vi "main.vi"() -> ()   [LabVIEW 2022 SP3]
uses:
  message.ctl
  states.ctl
  operationTypes.ctl
  consumer_data_structure.ctl
  <vilib>/picture/picture.llb/imagedata.ctl
  <vilib>/picture/picture.llb/Draw True-Color Pixmap.vi
panel:
  in  "Sharpen":bool
  in  "Filter":bool
  in  "Blur":bool
  out "Processed image":picture
  out "Input image":picture
  in  "stop":bool
  in  "Image path":path
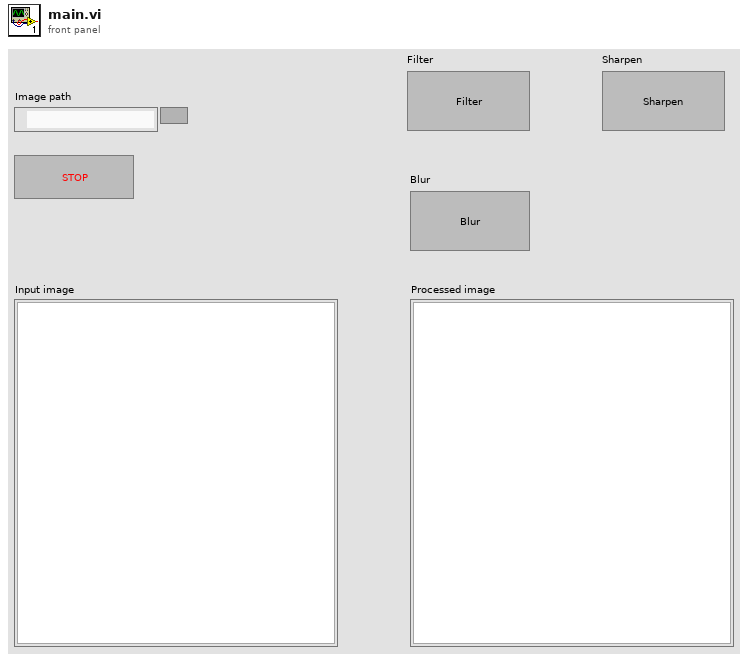
[diagram p1: front panel]
types:
  T1 = typedef "message.ctl" = cluster{"Command":T2, "data":variant}
  T2 = typedef "states.ctl" = enum16{"ErrorDefault", "Init", "ReadImage", "ProcessImage", "Stop"}
  T3 = typedef "operationTypes.ctl" = enum16{"Blur", "Sharpen", "Filter"}
  T4 = typedef "imagedata.ctl" = cluster{"image type":i32, "image depth":i32, "image":u8[], "mask":u8[], "colors":u32[], "Rectangle":cluster{"left":i16, "top":i16, "right":i16, "bottom":i16}}
  T5 = typedef "consumer_data_structure.ctl" = cluster{"Processed image":T4, "Input image":T4}
  T6 = typedef "LVBoundsTypeDef.ctl" = cluster{"Width":u32, "Height":u32}
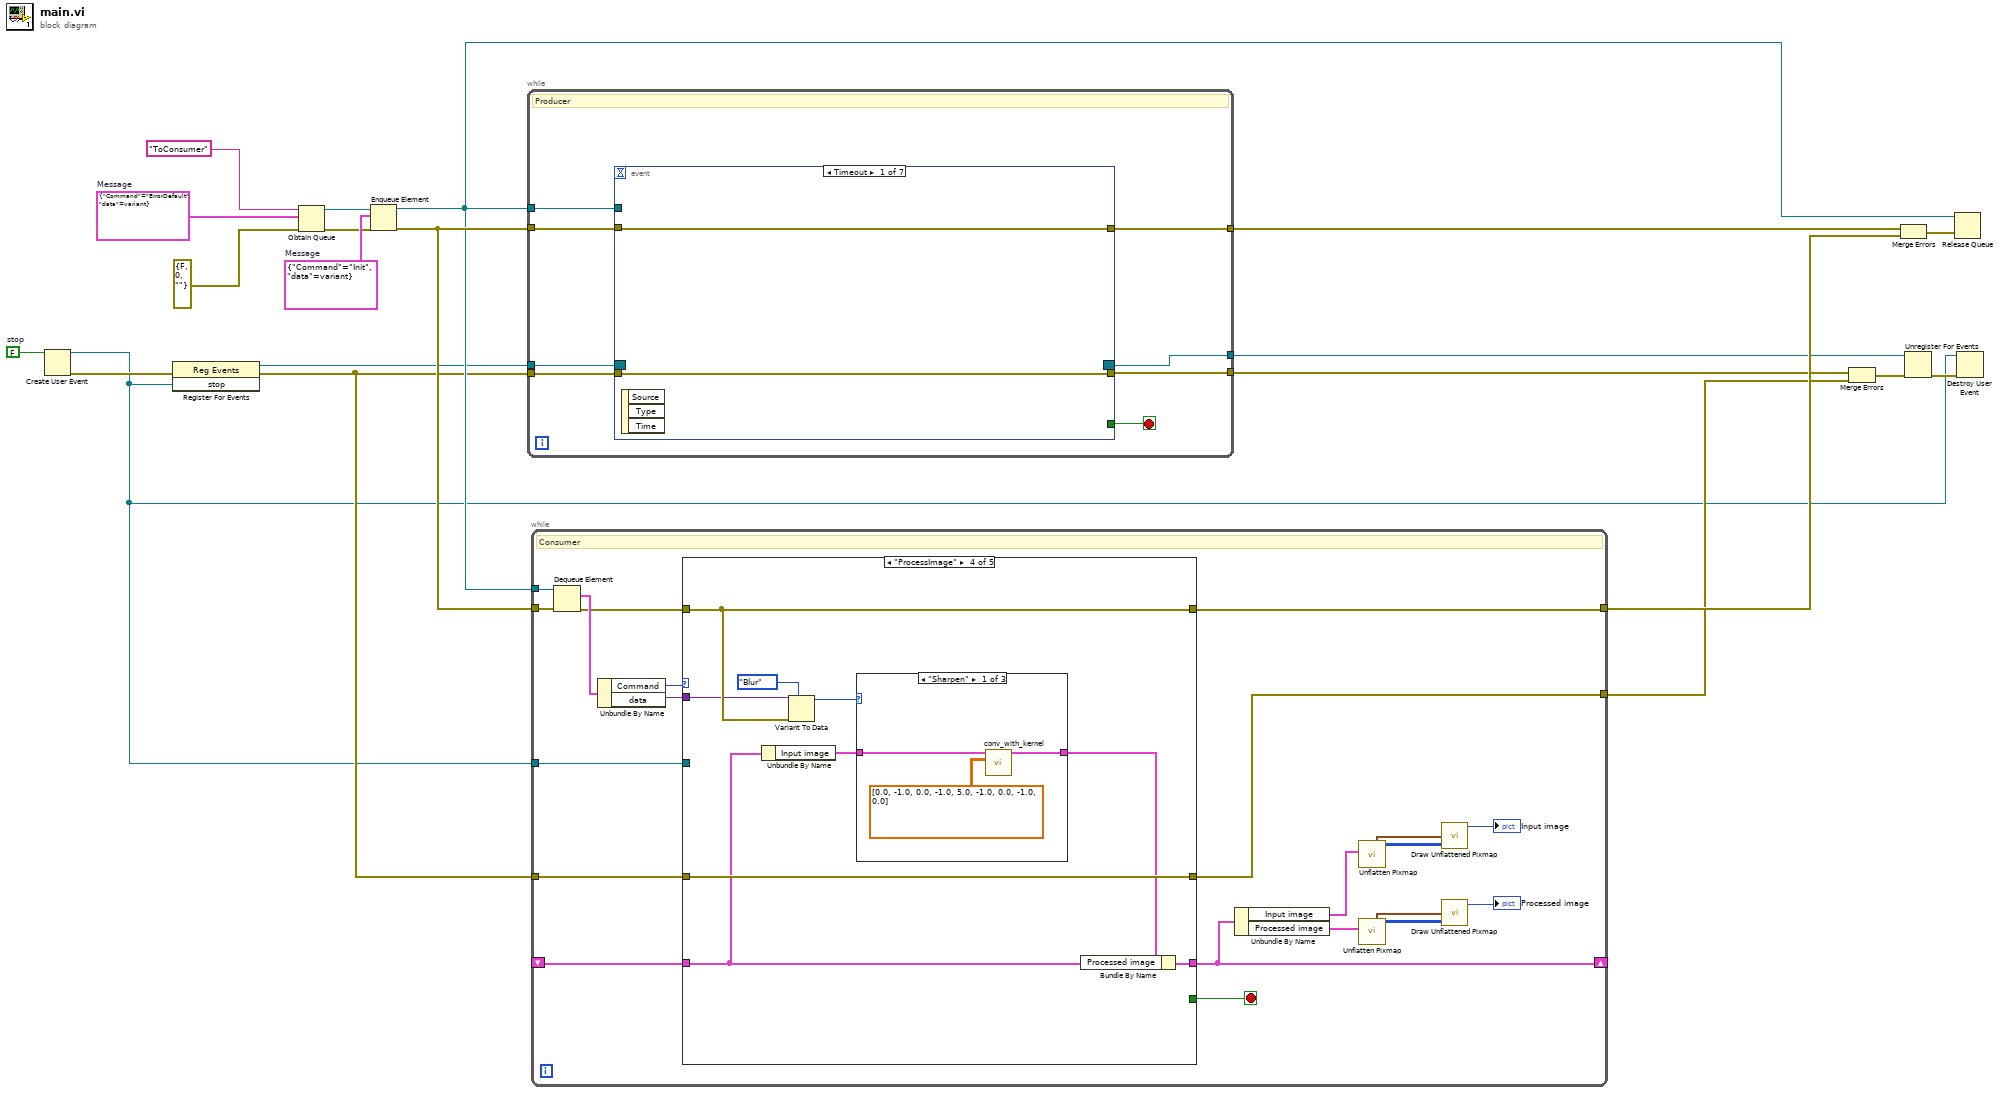
[diagram p0: block diagram]
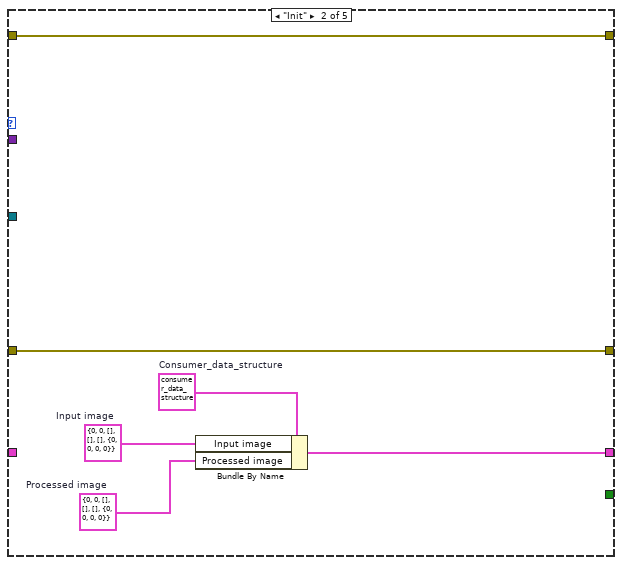
[diagram p3: hidden frame]
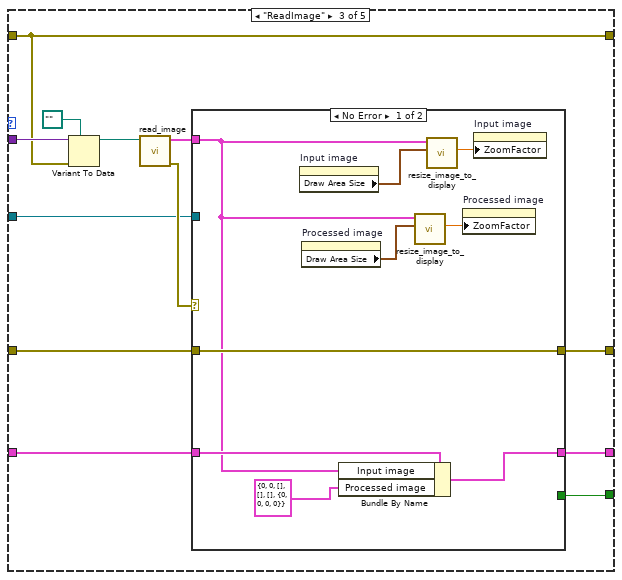
[diagram p4: hidden frame]
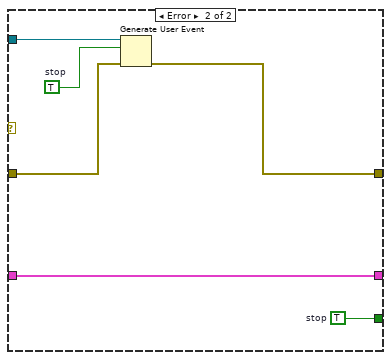
[diagram p5: hidden frame]
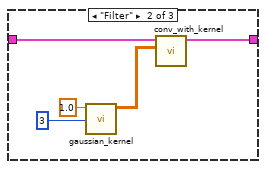
[diagram p6: hidden frame]
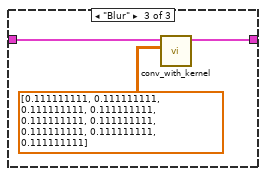
[diagram p7: hidden frame]
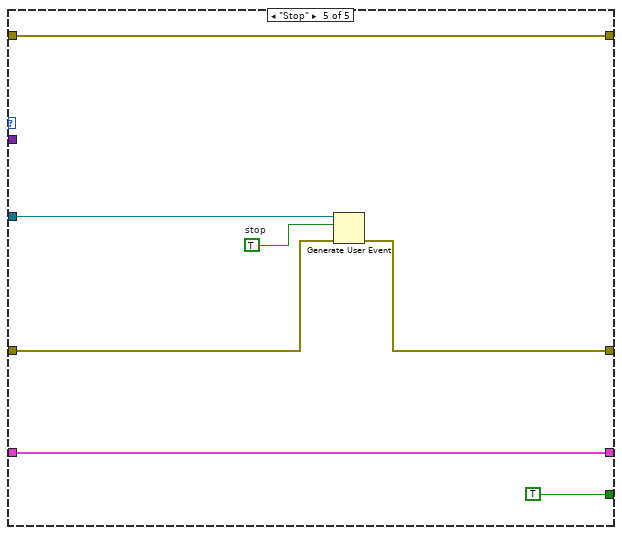
[diagram p8: hidden frame]
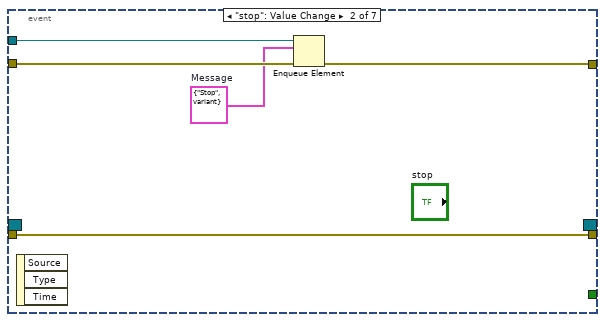
[diagram p9: hidden frame]
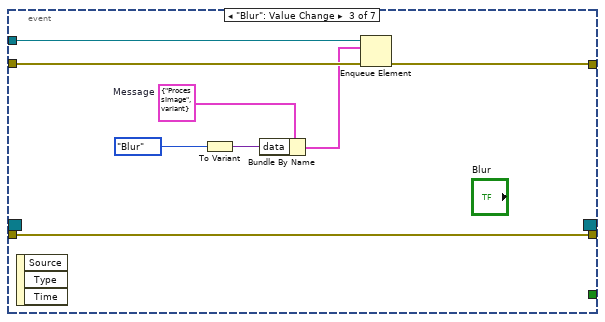
[diagram p10: hidden frame]
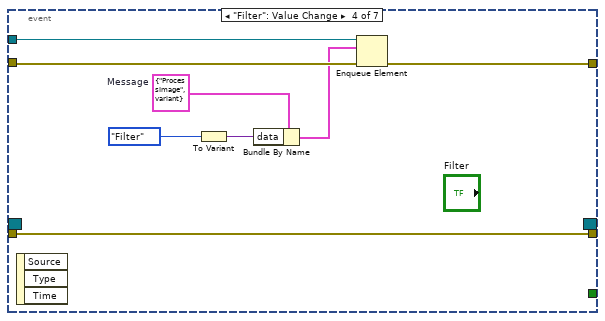
[diagram p11: hidden frame]
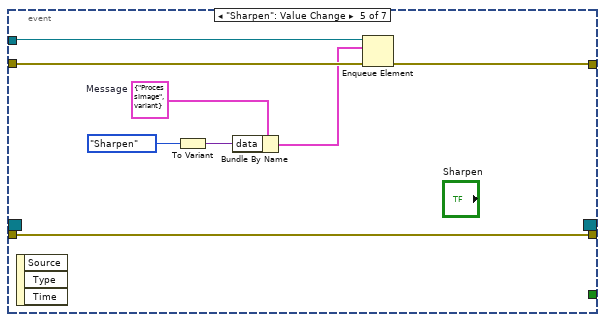
[diagram p12: hidden frame]
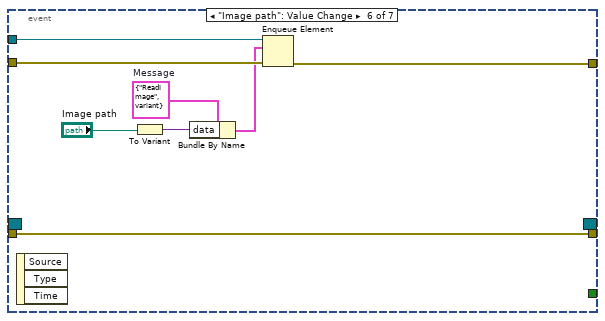
[diagram p13: hidden frame]
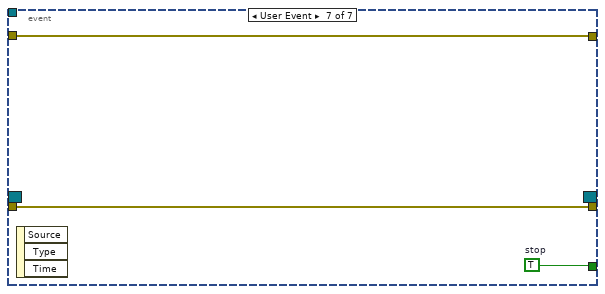
[diagram p14: hidden frame]
diagram:
  w10 = FALSE  # stop
  w18 = T1 {"Command"=enum."Init", "data"=variant(cluster{"Image path":path} {"Image path"=path ""})}  # Message
  w20 = T1 {"Command"=enum."ErrorDefault", "data"=variant(cluster{"Image path":path} {"Image path"=path ""})}  # Message
  n1 = Create User Event(user event datatype=w10) -> (user event=w1:refnum<user-event>, error out=w9:errorcluster)  [unwired: 1 in]
  n2 = register-events(error in=w9, w1) -> (reference out=w8:refnum<event-registration>, error out=w4:errorcluster)  [unwired: 1 in]
  n3 = Obtain Queue(name (unnamed)="ToConsumer", element data type=w20, error in (no error)=errorcluster {"status"=FALSE, "code"=0, "source"=""}) -> (queue out=w19:refnum<queue>, error out=w16:errorcluster)  [unwired: 2 in, 1 out]
  n4 = Enqueue Element(queue=w19, element=w18, error in (no error)=w16) -> (queue out=w11:refnum<queue>, error out=w15:errorcluster)  [unwired: 1 in, 1 out]
  n5 = while "Producer" {
    tunnel: w11 -> [w29]
    tunnel: w15 -> [w28]
    tunnel: [w27] -> w13
    tunnel: w8 -> [w25]
    tunnel: [w24] -> w6
    tunnel: w4 -> [w23]
    tunnel: [w22] -> w2
    stop <- w26 stop-if-true
    # "Producer"
    n6 = event shown="[0] Timeout" {
      selector: w25 -> [_ _ _ _ _ _ _]
      dyn-events: [_ _ _ _ _ _ _] -> w24
      timeout: _ -> [_ _ _ _ _ _ _]
      tunnel: w29 -> [_ w36 w44 w52 w60 w68 _]
      tunnel: w28 -> [w31 w35 w43 w51 w59 w67 w69]
      tunnel: [w31 w32 w42 w50 w58 w64 w69] -> w27
      tunnel: [_ _ _ _ _ _ w71] -> w26
      tunnel: w23 -> [w30 w33 w41 w49 w57 w63 w70]
      tunnel: [w30 w33 w41 w49 w57 w63 w70] -> w22
      event Timeout {
        n7 = event-data() -> ()  [unwired: 1 in, 3 out]
      }
      event "stop": Value Change {
        w34 = T1 {"Command"=enum."Stop", "data"=variant(cluster{"Image path":path} {"Image path"=path ""})}  # Message
        n8 = event-data() -> ()  [unwired: 1 in, 3 out]
        n9 = Enqueue Element(queue=w36, element=w34, error in (no error)=w35) -> (error out=w32:errorcluster)  [unwired: 1 in, 2 out]
      }
      event "Blur": Value Change {
        w38 = T1 {"Command"=enum."ProcessImage", "data"=variant(cluster{"Image path":path} {"Image path"=path ""})}  # Message
        n10 = event-data() -> ()  [unwired: 1 in, 3 out]
        n11 = To Variant(anything=operationTypes."Blur") -> (Variant=w40:variant)
        n12 = Bundle By Name(cluster=w38, "data"=w40) -> (w37:T1)
        n13 = Enqueue Element(queue=w44, element=w37, error in (no error)=w43) -> (error out=w42:errorcluster)  [unwired: 1 in, 2 out]
      }
      event "Filter": Value Change {
        w46 = T1 {"Command"=enum."ProcessImage", "data"=variant(cluster{"Image path":path} {"Image path"=path ""})}  # Message
        n14 = event-data() -> ()  [unwired: 1 in, 3 out]
        n15 = To Variant(anything=operationTypes."Filter") -> (Variant=w48:variant)
        n16 = Bundle By Name(cluster=w46, "data"=w48) -> (w45:T1)
        n17 = Enqueue Element(queue=w52, element=w45, error in (no error)=w51) -> (error out=w50:errorcluster)  [unwired: 1 in, 2 out]
      }
      event "Sharpen": Value Change {
        w54 = T1 {"Command"=enum."ProcessImage", "data"=variant(cluster{"Image path":path} {"Image path"=path ""})}  # Message
        n18 = event-data() -> ()  [unwired: 1 in, 3 out]
        n19 = To Variant(anything=operationTypes."Sharpen") -> (Variant=w56:variant)
        n20 = Bundle By Name(cluster=w54, "data"=w56) -> (w53:T1)
        n21 = Enqueue Element(queue=w60, element=w53, error in (no error)=w59) -> (error out=w58:errorcluster)  [unwired: 1 in, 2 out]
      }
      event "Image path": Value Change {
        w66 = T1 {"Command"=enum."ReadImage", "data"=variant(cluster{"Image path":path} {"Image path"=path ""})}  # Message
        n22 = event-data() -> ()  [unwired: 1 in, 3 out]
        n23 = To Variant(anything="Image path") -> (Variant=w61:variant)
        n24 = Bundle By Name(cluster=w66, "data"=w61) -> (w65:T1)
        n25 = Enqueue Element(queue=w68, element=w65, error in (no error)=w67) -> (error out=w64:errorcluster)  [unwired: 1 in, 2 out]
      }
      event User Event {
        w71 = TRUE  # stop
        n26 = event-data() -> ()  [unwired: 1 in, 3 out]
      }
    }
  }
  n27 = while "Consumer" {
    tunnel: w11 -> [w92]
    tunnel: w15 -> [w91]
    shift-right: [w83] -> _
    shift-left: _ -> [w88]
    tunnel: [w85] -> w14
    tunnel: w1 -> [w82]
    tunnel: w4 -> [w81]
    tunnel: [w80] -> w3
    stop <- w84 stop-if-true
    # "Consumer"
    n28 = Dequeue Element(queue=w92, error in (no error)=w91) -> (element=w90:T1, error out=w86:errorcluster)  [unwired: 1 in, 2 out]
    n29 = Unbundle By Name(w90) -> ("Command"=w89:T2, "data"=w87:variant)
    n30 = case shown="\"ProcessImage\"" w89 {
      tunnel: [w94 w100 w112 w130 w153] -> w83
      tunnel: w88 -> [w94 _ w113 w131 w153]
      tunnel: w87 -> [_ _ w105 w135 _]
      tunnel: [w95 w99 w103 w136 w154] -> w85
      tunnel: w86 -> [w95 w99 w103 w136 w154]
      tunnel: [_ _ w106 _ TRUE] -> w84
      tunnel: w82 -> [_ _ w109 _ w149]
      tunnel: w81 -> [w93 w98 w108 w137 w151]
      tunnel: [w93 w98 w107 w137 w150] -> w80
      frame "ErrorDefault", Default {
      }
      frame "Init" {
        w96 = T4 {"image type"=0, "image depth"=0, "image"=[], "mask"=[], "colors"=[], "Rectangle"={"left"=0, "top"=0, "right"=0, "bottom"=0}}  # Processed image
        w97 = T4 {"image type"=0, "image depth"=0, "image"=[], "mask"=[], "colors"=[], "Rectangle"={"left"=0, "top"=0, "right"=0, "bottom"=0}}  # Input image
        w101 = T5 {"Processed image"={"image type"=0, "image depth"=0, "image"=[], "mask"=[], "colors"=[], "Rectangle"={"left"=0, "top"=0, "right"=0, "bottom"=0}}, "Input image"={"image type"=0, "image depth"=0, "image"=[], "mask"=[], "colors"=[], "Rectangle"={"left"=0, "top"=0, "right"=0, "bottom"=0}}}  # Consumer_data_structure
        n31 = Bundle By Name(cluster=w101, "Input image"=w97, "Processed image"=w96) -> (w100:T5)
      }
      frame "ReadImage" {
        n32 = Variant To Data(error in=w103, type=path "", Variant=w105) -> (data=w102:path)  [unwired: 1 out]
        n33 = call "read_image.vi"("Image Path"=w102) -> ("error out"=w110:errorcluster, "Output image"=w111:T4)  [unwired: 9 in]
        n34 = case shown="No Error" w110 {
          tunnel: w113 -> [w118 w124]
          tunnel: [w117 w124] -> w112
          tunnel: w111 -> [w115 _]
          tunnel: w109 -> [_ w128]
          tunnel: w108 -> [w116 w127]
          tunnel: [w116 w125] -> w107
          tunnel: [_ w123] -> w106
          frame No Error {
            n35 = property on="Input image" class="Pict"() -> ("Draw Area Size"=w120:T6)  [unwired: 2 in, 2 out]
            n36 = property on="Processed image" class="Pict"() -> ("Draw Area Size"=w119:T6)  [unwired: 2 in, 2 out]
            n37 = Bundle By Name(cluster=w118, "Input image"=w115, "Processed image"=T4 {"image type"=0, "image depth"=0, "image"=[], "mask"=[], "colors"=[], "Rectangle"={"left"=0, "top"=0, "right"=0, "bottom"=0}}) -> (w117:T5)
            n38 = call "resize_image_to_display.vi"("DrawAreaSize"=w119, "image data"=w115) -> ("Zoom factor"=w121:dbl)  [unwired: 9 in]
            n39 = call "resize_image_to_display.vi"("DrawAreaSize"=w120, "image data"=w115) -> ("Zoom factor"=w122:dbl)  [unwired: 9 in]
            n40 = property on="Processed image" class="Pict"("ZoomFactor"=w121) -> ()  [unwired: 2 in, 2 out]
            n41 = property on="Input image" class="Pict"("ZoomFactor"=w122) -> ()  [unwired: 2 in, 2 out]
          }
          frame Error {
            w123 = TRUE  # stop
            w126 = TRUE  # stop
            n42 = Generate User Event(user event=w128, event data cluster=w126, error in=w127) -> (error out=w125:errorcluster)  [unwired: 1 in, 1 out]
          }
        }
      }
      frame "ProcessImage" {
        n43 = Unbundle By Name(w131) -> ("Input image"=w132:T4)
        n44 = Variant To Data(error in=w136, type=operationTypes."Blur", Variant=w135) -> (data=w133:T3)  [unwired: 1 out]
        n45 = case shown="\"Sharpen\"" w133 {
          tunnel: w132 -> [w140 w145 w148]
          tunnel: [w139 w144 w147] -> w129
          frame "Sharpen" {
            n46 = call "conv_with_kernel.vi"("Kernel"=dbl[][] [[0.0, -1.0, 0.0], [-1.0, 5.0, -1.0], [0.0, -1.0, 0.0]], "Image"=w140) -> ("Proccessed image"=w139:T4)  [unwired: 9 in]
          }
          frame "Filter" {
            n47 = call "gaussian_kernel.vi"("N"=3, "Sigma"=1.0) -> ("Gaussian kernel"=w143:dbl[][])  [unwired: 9 in]
            n48 = call "conv_with_kernel.vi"("Kernel"=w143, "Image"=w145) -> ("Proccessed image"=w144:T4)  [unwired: 9 in]
          }
          frame "Blur" {
            n49 = call "conv_with_kernel.vi"("Kernel"=dbl[][] [[0.111111111, 0.111111111, 0.111111111], [0.111111111, 0.111111111, 0.111111111], [0.111111111, 0.111111111, 0.111111111]], "Image"=w148) -> ("Proccessed image"=w147:T4)  [unwired: 9 in]
          }
        }
        n50 = Bundle By Name(cluster=w131, "Processed image"=w129) -> (w130:T5)
      }
      frame "Stop" {
        w152 = TRUE  # stop
        n51 = Generate User Event(user event=w149, event data cluster=w152, error in=w151) -> (error out=w150:errorcluster)  [unwired: 1 in, 1 out]
      }
    }
    n52 = Unbundle By Name(w83) -> ("Input image"=w77:T4, "Processed image"=w73:T4)
    n53 = call <vilib>:"Unflatten Pixmap.vi"("image data"=w77) -> ("24-bit pixmap"=w78:u32[][], "top left"=w79:cluster{"x":i16, "y":i16})  [unwired: 4 in, 5 out]
    n54 = call <vilib>:"Unflatten Pixmap.vi"("image data"=w73) -> ("24-bit pixmap"=w75:u32[][], "top left"=w76:cluster{"x":i16, "y":i16})  [unwired: 4 in, 5 out]
    n55 = call-poly <vilib>:"Draw Unflattened Pixmap.vi"("top left point(0, 0)"=w79, "data (RGB format)"=w78) -> ("new picture"=→"Input image":picture)  [unwired: 7 in]
    n56 = call-poly <vilib>:"Draw Unflattened Pixmap.vi"("top left point(0, 0)"=w76, "data (RGB format)"=w75) -> ("new picture"=→"Processed image":picture)  [unwired: 7 in]
  }
  n57 = Merge Errors(w2, w3) -> (w5:errorcluster)
  n58 = Merge Errors(w13, w14) -> (w12:errorcluster)
  n59 = Unregister For Events(event registration refnum=w6, error in=w5) -> (error out=w7:errorcluster)
  n60 = Release Queue(queue=w11, error in (no error)=w12) -> ()  [unwired: 1 in, 3 out]
  n61 = Destroy User Event(user event=w1, error in=w7) -> ()  [unwired: 1 out]
